vi "onDependencyStopped.vi"(8 "error in":errorcluster, 9 "Dependency":refnum<class "SMO.lvclass">, 11 "SMO in":refnum<class "SMO.lvclass">) -> (0 "error out":errorcluster, 3 "SMO out":refnum<class "SMO.lvclass">)   [LabVIEW 2021, in "smo.lvlib" / "SMO.lvclass"]
uses:
  SMO.lvclass
  SMO.lvclass/SMO.ctl
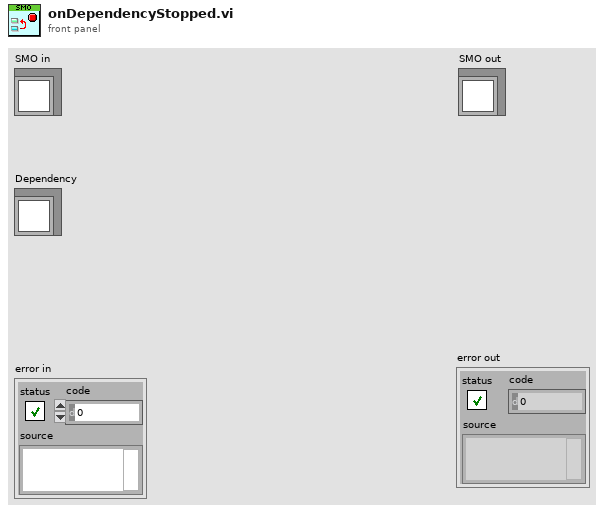
[diagram p1: front panel]
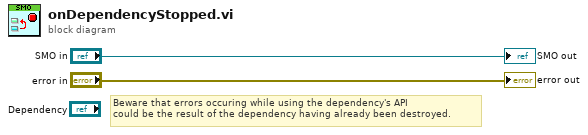
[diagram p0: block diagram]
diagram:
  # "Beware that errors occuring while using the dependency's API\ncould be the result of the dependency having already been destroyed."
  "SMO out" <- "SMO in"
  "error out" <- "error in"
